vi "Write Numeric Char.vi"(8 "error in (no error)":errorcluster, 10 "Numeric In":string, 11 "Character LCD in":refnum<class "LEDAlphaNumeric.lvclass">) -> (0 "error out":errorcluster, 3 "Character LCD out":refnum<class "LEDAlphaNumeric.lvclass">)   [LabVIEW 2020, in "CTI-Peripheral.lvlib" / "LEDAlphaNumeric.lvclass"]
uses:
  LEDAlphaNumeric.lvclass
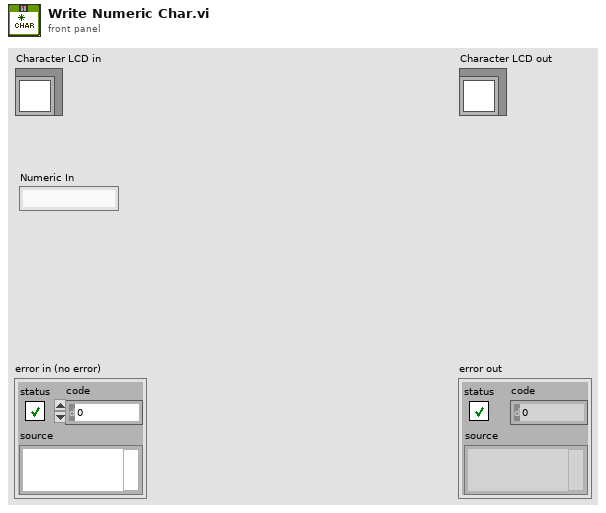
[diagram p1: front panel]
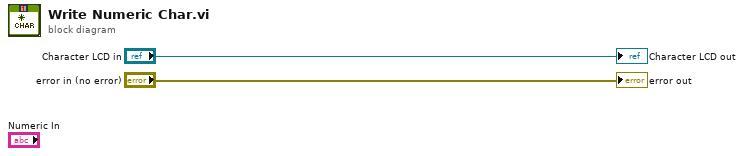
[diagram p0: block diagram]
diagram:
  "error out" <- "error in (no error)"
  "Character LCD out" <- "Character LCD in"
